vi "Dac_Output_cam_trig_synchronized_acquisition_updown.vi"(0 "Generate two signals":dbl[](graph)=array[10500 elements], 1 "Image acquisition time (ms)":dbl=76.0, 2 "Delay between frames (ms)":dbl=24.0) -> ()   [LabVIEW 2020]
uses:
  <vilib>/DAQmx/write.llb/DAQmx Write (Analog Wfm 1Chan NSamp).vi
  <vilib>/DAQmx/create/channels.llb/DAQmx Create Channel (AO-Voltage-Basic).vi
  <vilib>/DAQmx/configure/timing.llb/DAQmx Timing (Sample Clock).vi
  Global stop DAQ.vi
  <vilib>/DAQmx/miscellaneous.llb/DAQmx Fill In Error Info.vi
  <vilib>/DAQmx/create/channels.llb/DAQmx Create Channel (CO-Pulse Generation-Frequency).vi
  <vilib>/DAQmx/configure/timing.llb/DAQmx Timing (Implicit).vi
  <vilib>/DAQmx/configure/trigger.llb/DAQmx Start Trigger (Digital Edge).vi
  Global DAQ started.vi
  Global Counter count.vi
  Camera software flag.vi
  <resource>/objmgr/daqmx.rc
panel:
  out "Delay between frames (ms) 2":dbl=24.0
  out "Numeric":i32=67
  out "CO.Count":u32=1
  in  "Setup":enum16{"Test setup", "Microscope"}(ring)=enum."Microscope"
  out "error out 4":errorcluster={"status"=TRUE, "code"=-200488, "source"="DAQmx Stop Task.vi:3590031<append>\n"}
  out "error out 3":errorcluster
  in  "error in":errorcluster
  out "# Samples written per channel":u32=10500
  out "actual frequency":dbl=10000.0
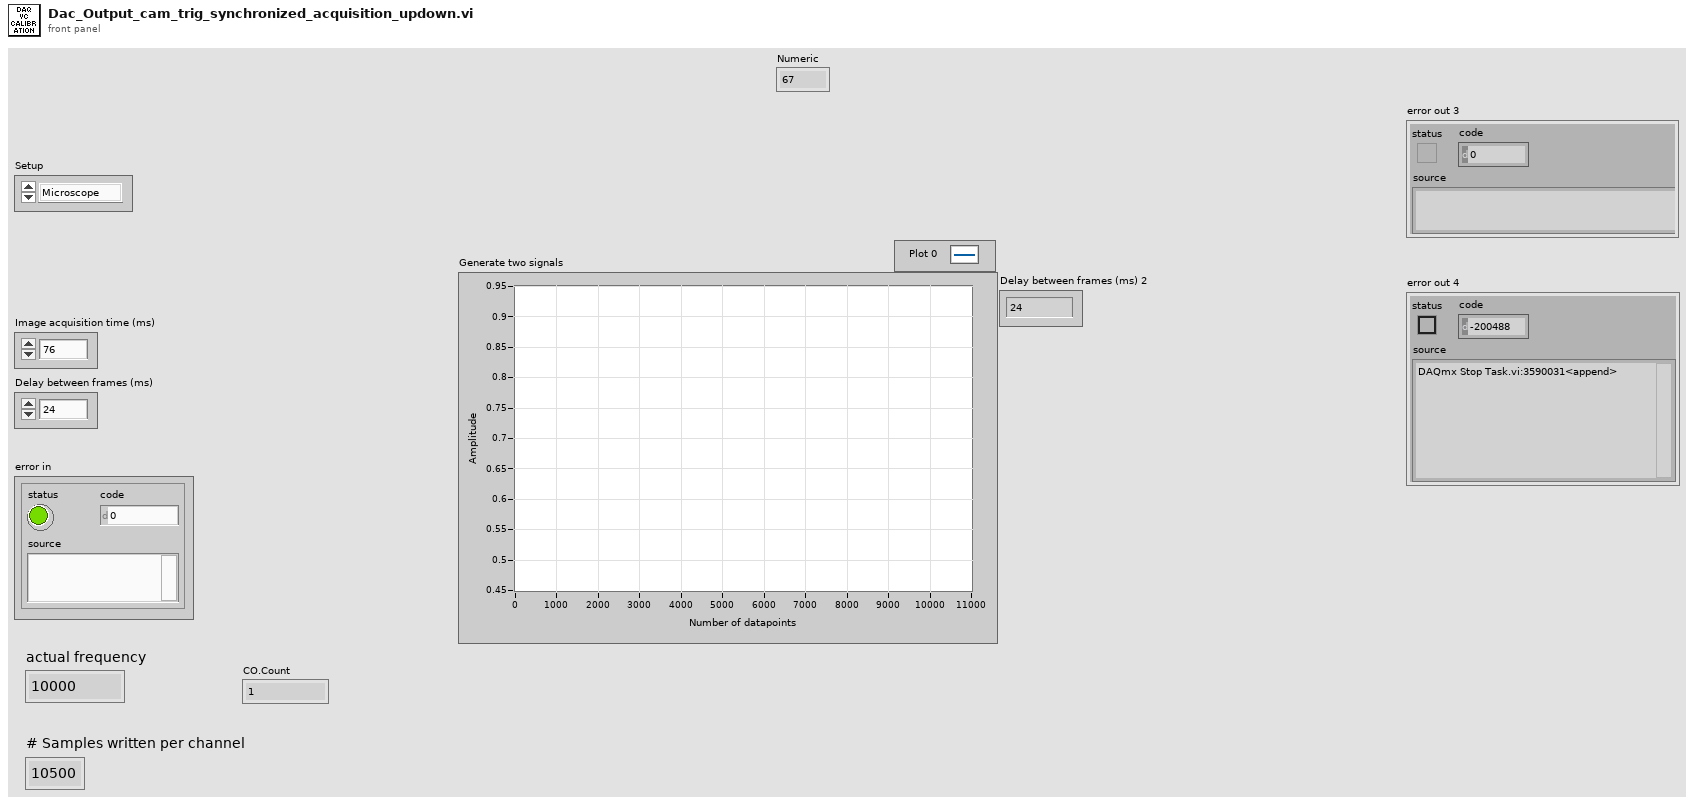
[diagram p1: front panel]
types:
  T1 = typedef "DAQ_channel_typedef.ctl" = cluster{"CO.Pulse.Term":tag, "Voice coil analog output":tag, "counter":tag, "CO.Pulse.Term 2":tag, "AOTF lines":tag, "counter 2":tag, "CO.Pulse.Term 3":tag, "counter 3":tag}
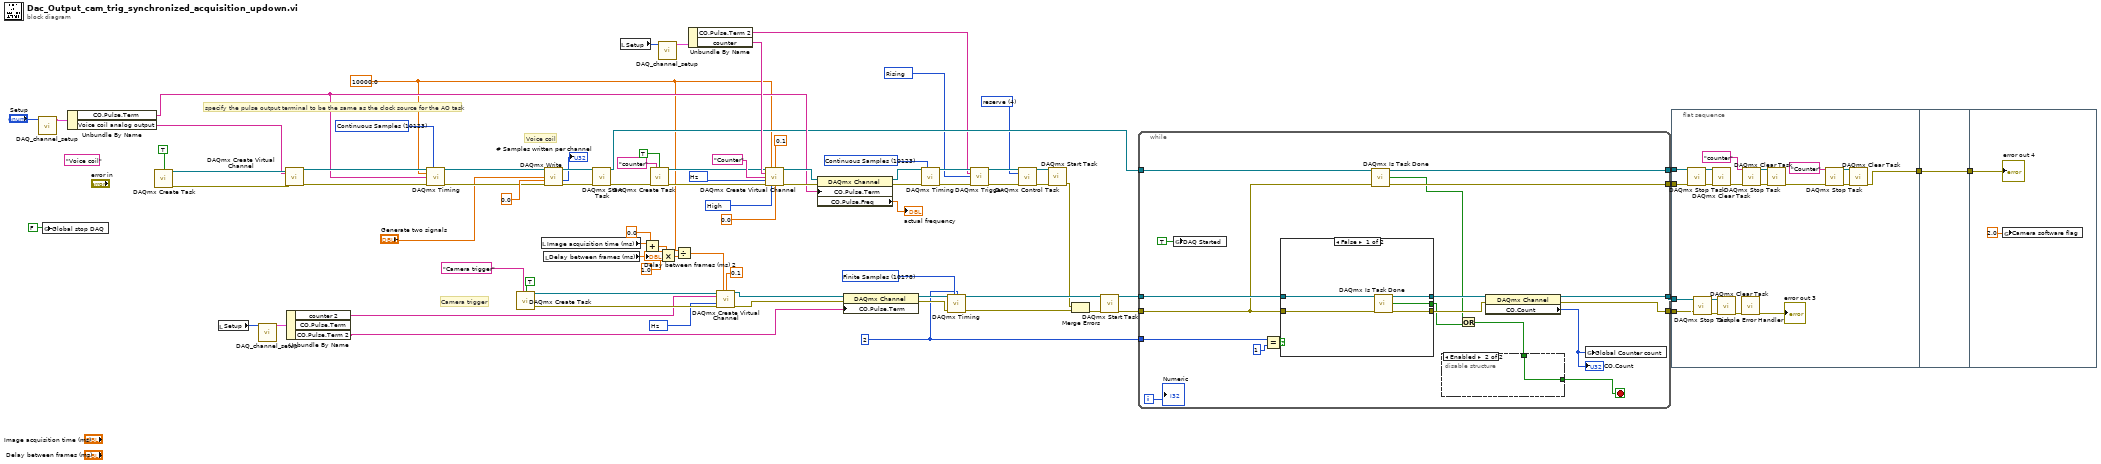
[diagram p0: block diagram]
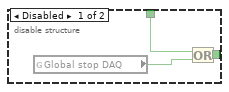
[diagram p2: hidden frame]
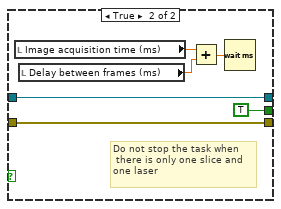
[diagram p3: hidden frame]
diagram:
  w9 = 2
  w16 = 4 items=["verify"=2, "reserve"=4, "commit"=3, "unreserve"=5, "abort"=6] ("action")
  w20 = 10280 items=["Rising"=10280, "Falling"=10171] ("edge")
  w26 = 10373 items=["Hz"=10373] ("units")
  (unwired) "Voice coil" ("new task name")
  w59 = 10178 items=["Finite Samples"=10178, "Continuous Samples"=10123, "Hardware Timed Single Point"=12522] ("sample mode")
  w70 = 10192 items=["High"=10192, "Low"=10214] ("idle state")
  w71 = 10373 items=["Hz"=10373] ("units")
  w64 = 10123 items=["Finite Samples"=10178, "Continuous Samples"=10123, "Hardware Timed Single Point"=12522] ("sample mode")
  w25 = 10000.0 ("rate")
  w81 = 10123 items=["Finite Samples"=10178, "Continuous Samples"=10123, "Hardware Timed Single Point"=12522] ("sample mode")
  # "Voice coil"
  # "Camera trigger"
  # "specify the pulse output terminal to be the same as the clock source for the AO task"
  n1 = call "DAQ_channel_setup.vi"("Text Ring"="Setup") -> ("DAQ channels OUT"=w42:T1)  [unwired: 10 in]
  n2 = global write "Global stop DAQ.vi" "Global stop DAQ"(FALSE ("Global stop DAQ")) -> ()
  n3 = Unbundle By Name(w42) -> ("CO.Pulse.Term"=w31:tag, "Voice coil analog output"=w43:tag)
  n4 = call <vilib>:"DAQmx Create Task.vi"("auto cleanup"=TRUE) -> ("task out"=w54:refnum<k21>, "error out"=w53:errorcluster)  [unwired: 13 in]
  n5 = local read "Setup"() -> (w36:enum16{"Test setup", "Microscope"})
  n6 = call "DAQ_channel_setup.vi"("Text Ring"=w36) -> ("DAQ channels OUT"=w39:T1)  [unwired: 10 in]
  n7 = call-poly <vilib>:"DAQmx Create Virtual Channel.vi"("task in"=w54, "physical channels"=w43, "error in"=w53) -> ("task out"=w83:refnum<k21>, "error out"=w82:errorcluster)  [unwired: 11 in]
  n8 = Unbundle By Name(w39) -> ("counter 2"=w38:tag, "CO.Pulse.Term 2"=w10:tag)  [unwired: 1 out]
  n9 = call-poly <vilib>:"DAQmx Timing.vi"("task/channels in"=w83, "sample mode"=w81, "rate"=w25, "source"=w31, "error in"=w82) -> ("task out"=w66:refnum<k21>, "error out"=w65:errorcluster)  [unwired: 9 in]
  n10 = call <vilib>:"DAQmx Create Task.vi"("new task name"="Camera trigger", "auto cleanup"=TRUE) -> ("task out"=w51:refnum<k21>, "error out"=w52:errorcluster)  [unwired: 12 in]
  n11 = local read "Image acquisition time (ms)"() -> (w55:dbl)
  n12 = local read "Delay between frames (ms)"() -> (→"Delay between frames (ms) 2":dbl)
  n13 = call-poly <vilib>:"DAQmx Write.vi"("task/channels in"=w66, "data"="Generate two signals", "timeout"=0.0, "error in"=w65) -> ("task out"=w75:refnum<k21>, "number of samples written per channel"=→"# Samples written per channel":u32, "error out"=w74:errorcluster)  [unwired: 9 in]
  n14 = call <vilib>:"DAQmx Start Task.vi"("task/channels in"=w75, "error in"=w74) -> ("task out"=w30:refnum<k21>, "error out"=w69:errorcluster)  [unwired: 12 in]
  n15 = local read "Setup"() -> (w35:enum16{"Test setup", "Microscope"})
  n16 = Add(x=w55, y=0.0) -> (x+y=w7:dbl)
  n17 = call <vilib>:"DAQmx Create Task.vi"("new task name"="counter", "auto cleanup"=TRUE, "error in"=w69) -> ("task out"=w32:refnum<k21>, "error out"=w80:errorcluster)  [unwired: 11 in]
  n18 = call "DAQ_channel_setup.vi"("Text Ring"=w35) -> ("DAQ channels OUT"=w41:T1)  [unwired: 10 in]
  n19 = Multiply(x=w7, y=1.0) -> (x*y=w6:dbl)
  n20 = Divide(x=w25, y=w6) -> (x/y=w28:dbl)
  n21 = Unbundle By Name(w41) -> ("CO.Pulse.Term 2"=w19:tag, "counter"=w40:tag)
  n22 = call-poly <vilib>:"DAQmx Create Virtual Channel.vi"("task in"=w51, "frequency"=w28, "duty cycle"=0.1, "counter"=w38, "units"=w26, "error in"=w52) -> ("task out"=w63:refnum<k21>, "error out"=w57:errorcluster)  [unwired: 8 in]
  n23 = call-poly <vilib>:"DAQmx Create Virtual Channel.vi"("task in"=w32, "frequency"=w25, "duty cycle"=0.1, "counter"=w40, "name to assign"="Counter", "units"=w71, "error in"=w80, "idle state"=w70, "initial delay"=0.0) -> ("task out"=w79:refnum<k21>, "error out"=w78:errorcluster)  [unwired: 5 in]
  n24 = property class="DAQmx Channel"(reference=w79, error in=w78, "CO.Pulse.Term"=w31) -> (reference out=w76:refnum<k21>, error out=w77:errorcluster, "CO.Pulse.Freq"=→"actual frequency":dbl)
  n25 = property class="DAQmx Channel"(reference=w63, error in=w57, "CO.Pulse.Term"=w10) -> (reference out=w56:refnum<k21>, error out=w60:errorcluster)
  n26 = call-poly <vilib>:"DAQmx Timing.vi"("task/channels in"=w76, "sample mode"=w64, "error in"=w77) -> ("task out"=w22:refnum<k21>, "error out"=w21:errorcluster)  [unwired: 11 in]
  n27 = call-poly <vilib>:"DAQmx Timing.vi"("task/channels in"=w56, "sample mode"=w59, "samples per channel"=w9, "error in"=w60) -> ("task out"=w58:refnum<k21>, "error out"=w11:errorcluster)  [unwired: 10 in]
  n28 = call-poly <vilib>:"DAQmx Trigger.vi"("task/channels in"=w22, "source"=w19, "edge"=w20, "error in"=w21) -> ("task out"=w18:refnum<k21>, "error out"=w17:errorcluster)  [unwired: 10 in]
  n29 = call <vilib>:"DAQmx Control Task.vi"("task/channels in"=w18, "action"=w16, "error in"=w17) -> ("task out"=w15:refnum<k21>, "error out"=w14:errorcluster)  [unwired: 11 in]
  n30 = call <vilib>:"DAQmx Start Task.vi"("task/channels in"=w15, "error in"=w14) -> ("error out"=w12:errorcluster)  [unwired: 12 in, 1 out]
  n31 = Merge Errors(w12, w11) -> (w13:errorcluster)
  n32 = call <vilib>:"DAQmx Start Task.vi"("task/channels in"=w58, "error in"=w13) -> ("task out"=w62:refnum<k21>, "error out"=w61:errorcluster)  [unwired: 12 in]
  n33 = while {
    tunnel: w30 -> [w102]
    tunnel: w62 -> [w101]
    tunnel: w61 -> [w87]
    tunnel: [w100] -> w45
    tunnel: [w99] -> w44
    tunnel: [w96] -> w47
    tunnel: [w94] -> w46
    tunnel: w9 -> [w90]
    i -> [w84]
    stop <- w91 stop-if-true
    n34 = global write "Global DAQ started.vi" "DAQ Started"(TRUE ("DAQ Started")) -> ()
    n35 = Equal?(x=w90, y=1) -> (x = y?=w88:bool)
    n36 = case shown="False" w88 {
      tunnel: w101 -> [w111 w117]
      tunnel: w87 -> [w110 w116]
      tunnel: [w109 w117] -> w97
      tunnel: [w108 w116] -> w95
      tunnel: [w107 TRUE ("task done?")] -> w92
      frame False {
        n37 = call <vilib>:"DAQmx Is Task Done.vi"("task/channels in"=w111, "error in"=w110) -> ("task out"=w109:refnum<k21>, "task done?"=w107:bool, "error out"=w108:errorcluster)  [unwired: 11 in]
      }
      frame True {
        # "Do not stop the task when\n there is only one slice and \none laser"
        n38 = local read "Image acquisition time (ms)"() -> (w113:dbl)
        n39 = local read "Delay between frames (ms)"() -> (w114:dbl)
        n40 = Add(x=w113, y=w114) -> (x+y=w112:dbl)
        n41 = Wait (ms)(milliseconds to wait=w112) -> ()  [unwired: 1 out]
      }
    }
    n42 = call <vilib>:"DAQmx Is Task Done.vi"("task/channels in"=w102, "error in"=w87) -> ("task out"=w100:refnum<k21>, "task done?"=w86:bool, "error out"=w99:errorcluster)  [unwired: 11 in]
    n43 = Or(x=w86, y=w92) -> (x .or. y?=w85:bool)
    n44 = disable-structure shown="Enabled" {
      disable-tunnel: [w104 w106] -> w91
      disable-tunnel: w85 -> [w103 w106]
      frame Disabled {
        n45 = global read "Global stop DAQ.vi" "Global stop DAQ"() -> (w105:bool)
        n46 = Or(x=w103, y=w105) -> (x .or. y?=w104:bool)
      }
      frame Enabled {
      }
    }
    n47 = property class="DAQmx Channel"(reference=w97, error in=w95) -> (reference out=w96:refnum<k21>, error out=w94:errorcluster, "CO.Count"=w93:u32)
    "CO.Count" <- w93
    n48 = global write "Global Counter count.vi" "Global Counter count"(w93) -> ()
    "Numeric" <- w84
  }
  n49 = flat-sequence {
    tunnel: w47 -> [w136]
    tunnel: w46 -> [w135]
    tunnel: w45 -> [w134]
    tunnel: w44 -> [w133]
    tunnel: [w118] -> w4
    tunnel: w4 -> [w137]
    tunnel: [w137] -> w3
    tunnel: w3 -> [w139]
    frame #0 {
      n50 = call <vilib>:"DAQmx Stop Task.vi"("task/channels in"=w134, "error in"=w133) -> ("task out"=w128:refnum<k21>, "error out"=w127:errorcluster)  [unwired: 12 in]
      n51 = call <vilib>:"DAQmx Stop Task.vi"("task/channels in"=w136, "error in"=w135) -> ("task out"=w131:refnum<k21>, "error out"=w132:errorcluster)  [unwired: 12 in]
      n52 = call <vilib>:"DAQmx Clear Task.vi"("task in"=w128, "error in"=w127) -> ("error out"=w124:errorcluster)  [unwired: 13 in]
      n53 = call <vilib>:"DAQmx Clear Task.vi"("task in"=w131, "error in"=w132) -> ("error out"=w130:errorcluster)  [unwired: 13 in]
      n54 = call <vilib>:"Simple Error Handler.vi"("error in (no error)"=w130) -> ("error out"=→"error out 3":errorcluster)  [unwired: 4 in, 4 out]
      n55 = call <vilib>:"DAQmx Stop Task.vi"("task/channels in"="counter" ("new task name"), "error in"=w124) -> ("task out"=w126:refnum<k21>, "error out"=w125:errorcluster)  [unwired: 12 in]
      n56 = call <vilib>:"DAQmx Clear Task.vi"("task in"=w126, "error in"=w125) -> ("error out"=w123:errorcluster)  [unwired: 13 in]
      n57 = call <vilib>:"DAQmx Stop Task.vi"("task/channels in"="Counter" ("new task name"), "error in"=w123) -> ("task out"=w120:refnum<k21>, "error out"=w121:errorcluster)  [unwired: 12 in]
      n58 = call <vilib>:"DAQmx Clear Task.vi"("task in"=w120, "error in"=w121) -> ("error out"=w118:errorcluster)  [unwired: 13 in]
    }
    frame #1 {
    }
    frame #2 {
      n59 = global write "Camera software flag.vi" "Camera software flag"(2.0 ("Camera software flag")) -> ()
      "error out 4" <- w139
    }
  }
